vi "FPGAmain_5160_old.vi"() -> ()   [LabVIEW 2013]
uses:
  <vilib>/eio/EIONode/EIONode.xnode
  <vilib>/Platform/TimedLoop/XDataNode/wakeup.ctl
  <vilib>/Platform/TimedLoop/XDataNode/XDNodeRunTimeDep.lvlib
  <vilib>/Platform/TimedLoop/XDataNode/nitl_modes.ctl
  <vilib>/Platform/TimedLoop/XDataNode/timing_clust.ctl
  <vilib>/Platform/TimedLoop/XDataNode/XDataNode.xnode
  <vilib>/rvi/DataTransferAndStorage/Container/XNode/niFpgaContainer.xnode
  <vilib>/rvi/FIFO/Fifo_Resource/nirvififoEmulationWrite.vi
  <vilib>/rvi/FIFO/Fifo_Resource/nirvififoEmulationRead.vi
  <vilib>/rvi/interface/RandomDataEmulation/nirviRandomDataFpgaMultiElementTemplate.vi
  FPGA/AcquireState.ctl
  <instrlib>/FlexRIO/Libraries/Helper VIs/Counters/NI FlexRIO Counters.lvlib
  <instrlib>/FlexRIO/Libraries/Helper VIs/NI FlexRIO Helper VIs.lvlib
  <vilib>/rvi/FIFO/Fifo_Resource/nirvififoEmulationP2P.vi
  <vilib>/rvi/eio/common/nirviEmuTemplateMethod_errors.vi
  <vilib>/rvi/interface/RandomDataEmulation/nirviRandomDataFpgaReadWriteTemplate.vi
  FPGA/DataMode.ctl
panel:
  out "num data 2nd loop":u32
  out "timeout counter":i32
  out "num read":u32
  out "num to clock fifo":u32
  in  "Samples Per Trigger":i32 min=1 step=1
  in  "Trigger simulated data":bool
  in  "simulated phase":fxp<+,64,64>
  out "DMA Timed Out?":bool
  in  "phase":fxp<+,64,64>
  in  "Mode":T1
  in  "User Command Commit":bool
  in  "User Command":u8
  out "User Command Idle":bool
  out "User Command Status":u8
  in  "User Data 0":u16
  in  "User Data 1":u8
  out "PLL Locked":bool
  out "User Error":bool
  out "Configured?":bool
  # "Configuration"
  # "Aqcuistion"
  # "Simulated IQ"
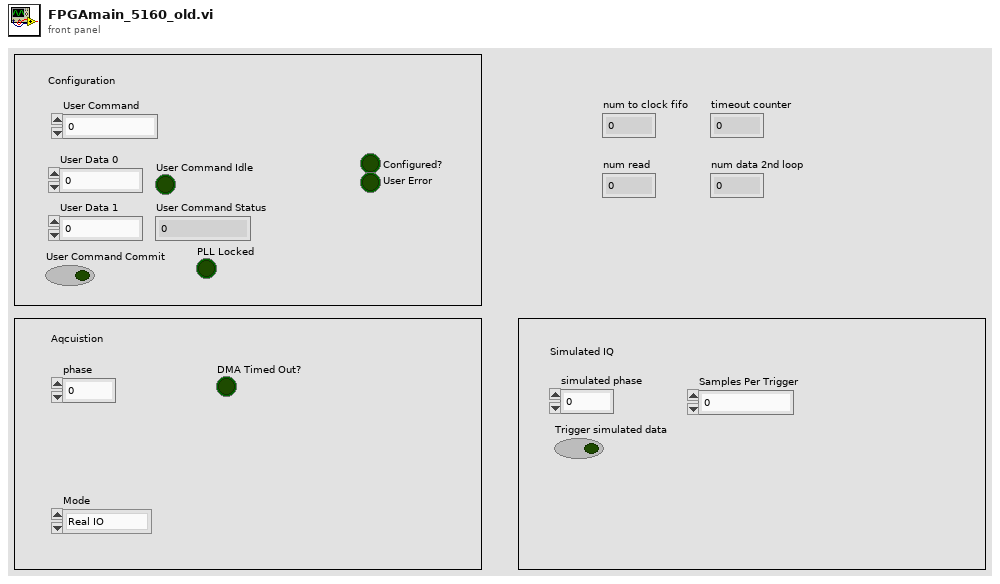
[diagram p1: front panel]
types:
  T1 = typedef "DataMode.ctl" = enum16{"Real IO", "Simulated"}
  T2 = typedef "AcquireState.ctl" = enum8{"Idle", "Acquire"}
  T3 = typedef "XDNodeRunTimeDep.lvlib/timing_clust.ctl" = cluster{"Expected End [f-1]":u64, "Actual End [f-1]":u64, "Finished Late? [f-1]":bool, "Expected End [i-1]":u64, "Actual End [i-1]":u64, "Finished Late? [i-1]":bool, "Expected Start [i]":u64, "Actual Start [i]":u64, "Expected Start [f]":u64, "Actual Start [f]":u64, "Source Name":string, "Structure Name":string, "Period":i64, "Deadline":i64, "Offset":i64, "Start":i64, "Priority":i32, "Timeout":i32, "Mode":T4, "Wakeup Reason":T5, "Error":errorcluster, "Source Type":string, "Secondary Source Type":string, "Global End Time":u64, "Global Start Time":u64, "Frame Duration":u64, "Iteration Duration":u64, "Assigned CPU":i32, "I/O Scan Engine Mode":u32}
  T4 = typedef "XDNodeRunTimeDep.lvlib/nitl_modes.ctl" = enum32{"No Change", "Process missed periods, maintain original phase", "Discard missed periods, maintain original phase", "Process missed periods, ignore original phase", "Discard missed periods, ignore original phase"}
  T5 = typedef "XDNodeRunTimeDep.lvlib/wakeup.ctl" = enum32{"Normal", "Aborted", "Asynchronous wakeup", "Timing source error", "Timed loop error", "Timeout"}
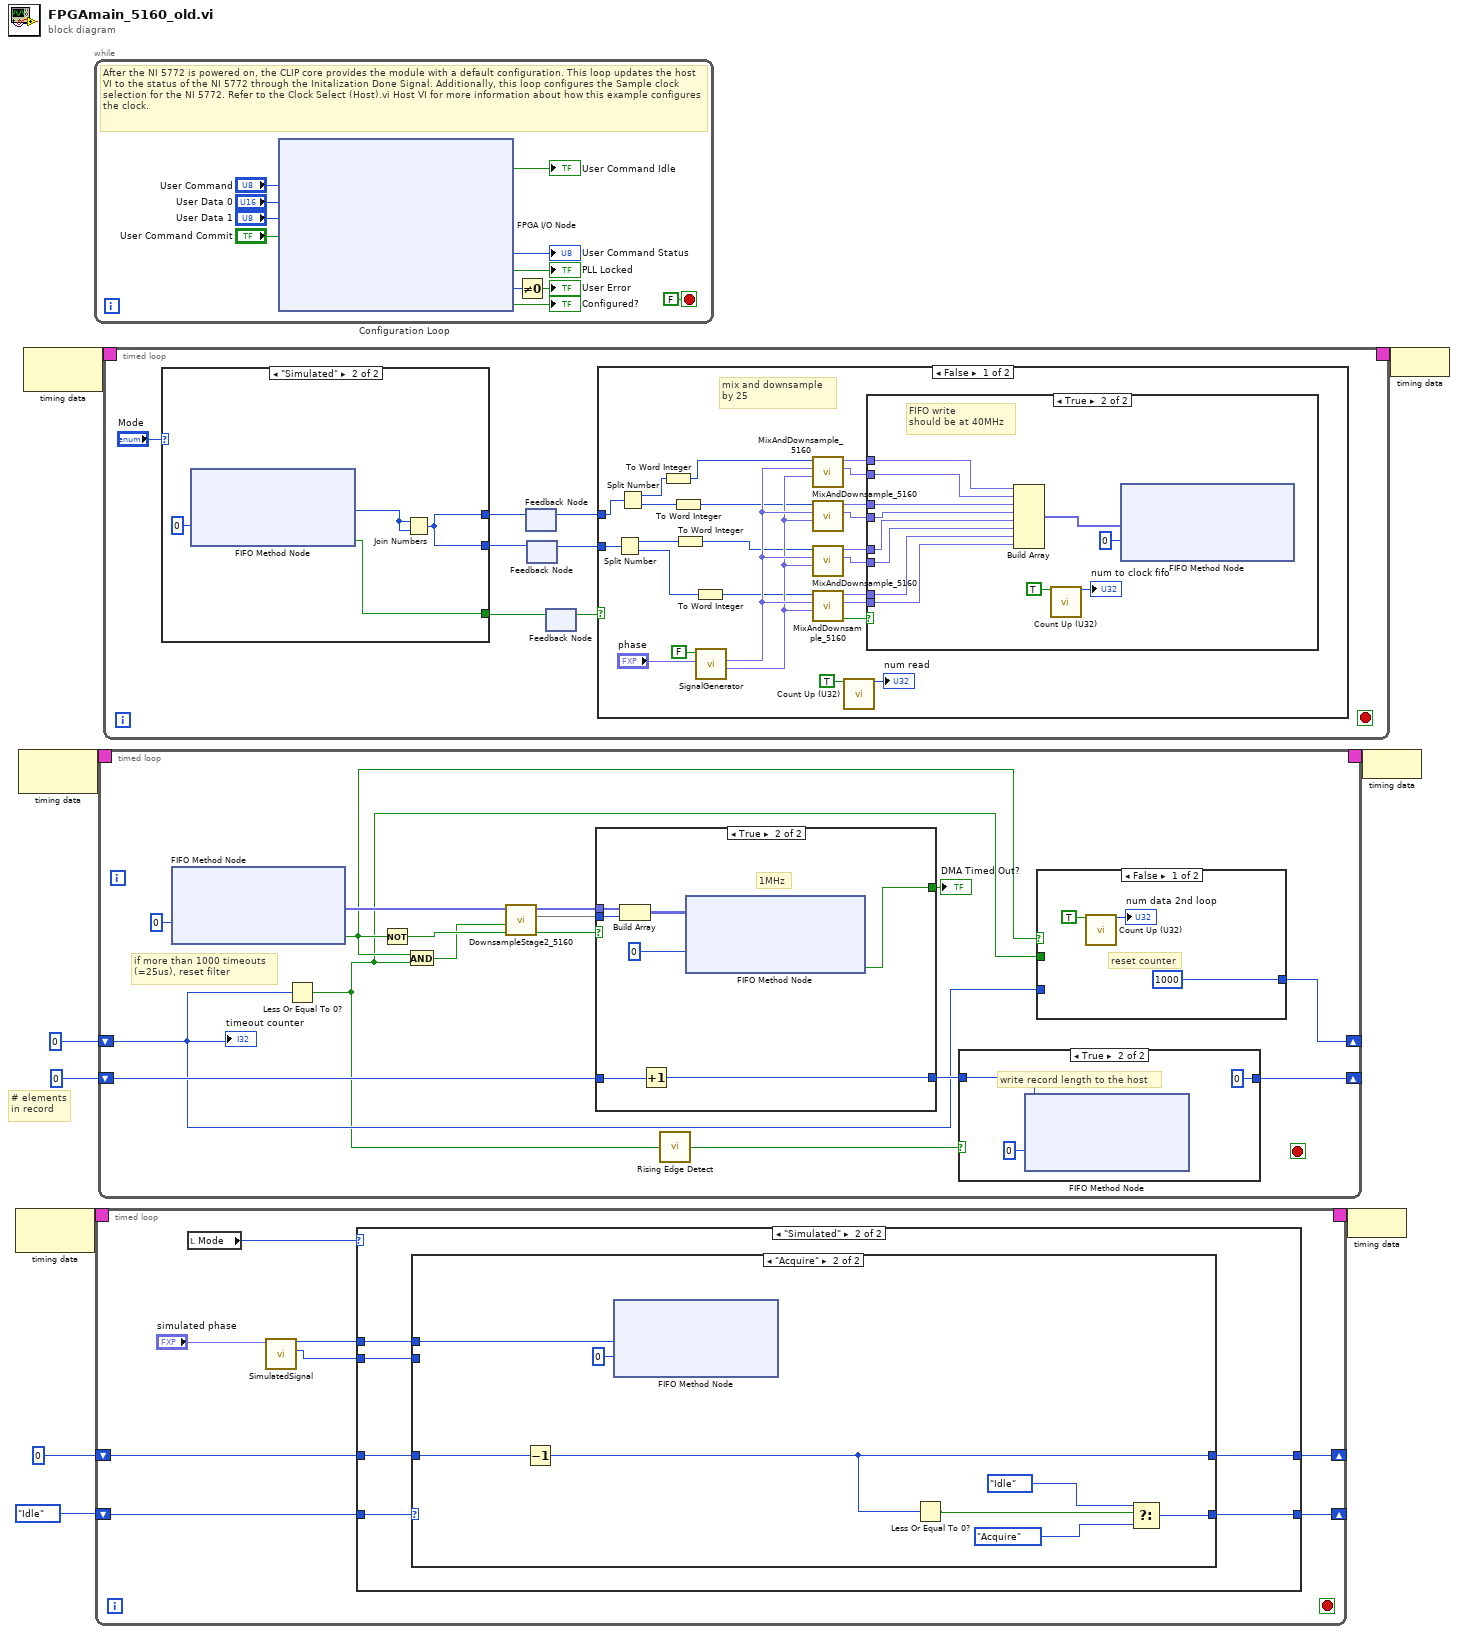
[diagram p0: block diagram]
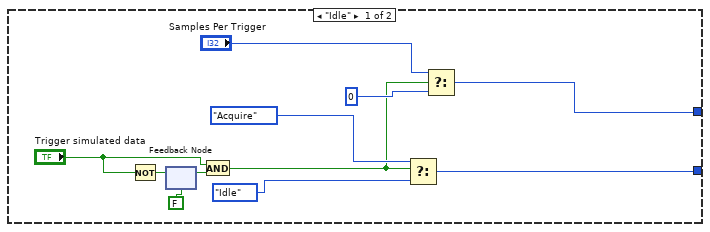
[diagram p3: hidden frame]
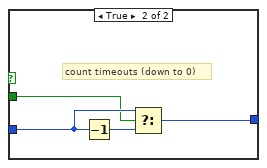
[diagram p4: hidden frame]
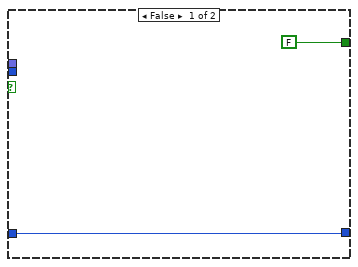
[diagram p6: hidden frame]
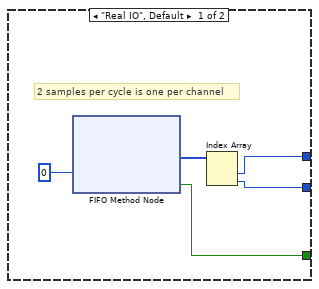
[diagram p9: hidden frame]
diagram:
  # "# elements\nin record"
  n1 = node-c288() -> (w6:T3)  [unwired: 1 in]
  n2 = node-c288() -> (w8:T3)  [unwired: 1 in]
  n3 = node-c288() -> (w10:T3)  [unwired: 1 in]
  n4 = while "Configuration Loop" {
    stop <- FALSE stop-if-true
    # "After the NI 5772 is powered on, the CLIP core provides the module with a default configuration. This loop updates the host VI to the status of the NI 5772 through the Initalization Done Signal. Additionally, this loop configures the Sample clock selection for the NI 5772. Refer to the Clock Select (Host).vi Host VI for more information about how this example configures the clock."
    n5 = xnode "FPGA I/O Node"("IO Module\\User Command"="User Command", "IO Module\\User Data 0"="User Data 0", "IO Module\\User Data 1"="User Data 1", "IO Module\\User Command Commit"="User Command Commit") -> ("IO Module\\User Command Idle"=→"User Command Idle":bool, "IO Module\\User Command Status"=→"User Command Status":u8, "IO Module\\PLL Locked"=→"PLL Locked":bool, "IO Module\\User Error"=w16:u8, "IO Module\\Initialization Done"=→"Configured?":bool)  [unwired: 9 in, 9 out]
    n6 = Not Equal To 0?(x=w16) -> (x != 0?=→"User Error":bool)
  }
  n7 = timed-loop {
    timing: w6 -> [_]
    timing-out: [_] -> w5
    shift-right: [w25] -> _
    shift-left: 0 ("f") -> [w24]
    shift-right: [w23] -> _
    shift-left: AcquireState."Idle" ("Acquire State") -> [w22]
    stop <- _ stop-if-true
    n8 = local read "Mode"() -> (w29:T1)
    n9 = call "SimulatedSignal.vi"("phase"="simulated phase") -> ("cos output"=w27:i16, "Sample output"=w28:i16)  [unwired: 9 in]
    n10 = case shown="\"Simulated\"" w29 {
      tunnel: w28 -> [_ w37]
      tunnel: w27 -> [_ w32]
      tunnel: [w31 w36] -> w25
      tunnel: w24 -> [w31 w35]
      tunnel: [w30 w34] -> w23
      tunnel: w22 -> [w30 w33]
      frame "Real IO" {
      }
      frame "Simulated" {
        n11 = case shown="\"Acquire\"" w33 {
          tunnel: w35 -> [_ w53]
          tunnel: [w42 w52] -> w34
          tunnel: [w39 w51] -> w36
          tunnel: w37 -> [_ w50]
          tunnel: w32 -> [_ _]
          frame "Idle" {
            n12 = Not(x="Trigger simulated data") -> (.not. x?=w43:bool)
            n13 = feedback #1(FALSE) -> (w44:bool)
            n14 = feedback-in #1(w43) -> ()
            n15 = And(x="Trigger simulated data", y=w44) -> (x .and. y?=w38:bool)
            n16 = Select(t=AcquireState."Acquire" ("Acquire State"), s=w38, f=AcquireState."Idle" ("Acquire State")) -> (s? t:f=w42:T2)
            n17 = Select(t="Samples Per Trigger", s=w38, f=0) -> (s? t:f=w39:i32)
          }
          frame "Acquire" {
            n18 = Decrement(x=w53) -> (x-1=w51:i32)
            n19 = xnode ("FIFO Method Node")("Element"=w50, "Timeout"=0) -> ()  [unwired: 1 in, 2 out]
            n20 = Less Or Equal To 0?(x=w51) -> (x <= 0?=w55:bool)
            n21 = Select(t=AcquireState."Idle" ("Acquire State"), s=w55, f=AcquireState."Acquire" ("Acquire State")) -> (s? t:f=w52:T2)
          }
        }
      }
    }
  }
  n22 = timed-loop {
    timing: w8 -> [_]
    timing-out: [_] -> w7
    shift-right: [w62] -> _
    shift-left: 0 ("y") -> [w61]
    shift-right: [w64] -> _
    shift-left: 0 ("y") -> [w66]
    stop <- _ stop-if-true
    # "if more than 1000 timeouts\n(=25us), reset filter"
    n23 = xnode ("FIFO Method Node")("Timeout"=0) -> ("Element"=w71:fxp<+/-,16,14>[], "Timed Out?"=w63:bool)  [unwired: 1 in, 1 out]
    n24 = Less Or Equal To 0?(x=w61) -> (x <= 0?=w60:bool)
    n25 = Not(x=w63) -> (.not. x?=w72:bool)
    n26 = And(x=w63, y=w60) -> (x .and. y?=w67:bool)
    n27 = call "DownsampleStage2_5160.vi"("valid in"=w72, "reset"=w67, "Element"=w71) -> ("valid out"=w73:bool, 2:w70, "Array"=w74:fxp<+/-,16,14>[])  [unwired: 6 in]
    n28 = case shown="True" w73 {
      tunnel: w74 -> [_ w93]
      tunnel: [FALSE ("Timed Out?") w91] -> w68
      tunnel: w70 -> [_ w92]
      tunnel: w66 -> [w86 w89]
      tunnel: [w86 w88] -> w65
      frame False {
      }
      frame True {
        # "1MHz"
        n29 = Build Array(w93, w92) -> (w90:fxp<+/-,16,14>[][])
        n30 = Increment(x=w89) -> (x+1=w88:i32)
        n31 = xnode ("FIFO Method Node")("Element"=w90, "Timeout"=0) -> ("Timed Out?"=w91:bool)  [unwired: 1 in, 1 out]
      }
    }
    "DMA Timed Out?" <- w68
    n32 = call <instrlib>:"Rising Edge Detect.vi"("signal"=w60) -> ("edge detected"=w59:bool)  [unwired: 14 in]
    n33 = case shown="True" w59 {
      tunnel: w65 -> [w82 w83]
      tunnel: [w82 0 ("y")] -> w64
      frame False {
      }
      frame True {
        # "write record length to the host"
        n34 = xnode ("FIFO Method Node")("Element"=w83, "Timeout"=0) -> ()  [unwired: 1 in, 2 out]
      }
    }
    n35 = case shown="False" w63 {
      tunnel: w60 -> [_ w79]
      tunnel: w61 -> [_ w80]
      tunnel: [1000 ("y") w78] -> w62
      frame False {
        # "reset counter"
        n36 = call <instrlib>:"Count Up (U32).vi"("increment"=TRUE) -> ("count out"=→"num data 2nd loop":u32)  [unwired: 14 in]
      }
      frame True {
        # "count timeouts (down to 0)"
        n37 = Decrement(x=w80) -> (x-1=w81:i32)
        n38 = Select(t=w80, s=w79, f=w81) -> (s? t:f=w78:i32)
      }
    }
    "timeout counter" <- w61
  }
  n39 = timed-loop {
    timing: w10 -> [_]
    timing-out: [_] -> w9
    stop <- _ stop-if-true
    n40 = case shown="\"Simulated\"" "Mode" {
      tunnel: [w143 w147] -> w102
      tunnel: [w141 w148] -> w99
      tunnel: [w142 w147] -> w98
      frame "Real IO", Default {
        # "2 samples per cycle is one per channel"
        n41 = xnode ("FIFO Method Node")("Timeout"=0) -> ("Element"=w145:u32[], "Timed Out?"=w141:bool)  [unwired: 1 in, 1 out]
        n42 = Index Array(array=w145) -> (element #1=w143:u32, element #2=w142:u32)  [unwired: 2 in]
      }
      frame "Simulated" {
        n43 = xnode ("FIFO Method Node")("Timeout"=0) -> ("Element"=w146:i16, "Timed Out?"=w148:bool)  [unwired: 1 in, 1 out]
        n44 = Join Numbers(hi=w146, lo=w146) -> ((hi.lo)=w147:u32)
      }
    }
    n45 = feedback-in #2(w102) -> ()
    n46 = feedback #2() -> (w101:u32)  [unwired: 1 in]
    n47 = feedback #3() -> (w97:u32)  [unwired: 1 in]
    n48 = feedback-in #3(w98) -> ()
    n49 = feedback #4() -> (w100:bool)  [unwired: 1 in]
    n50 = feedback-in #4(w99) -> ()
    n51 = case shown="False" w100 {
      tunnel: w101 -> [w119 _]
      tunnel: w97 -> [w108 _]
      frame False {
        # "mix and downsample\nby 25"
        n52 = Split Number(x=w108) -> (hi(x)=w109:u16, lo(x)=w110:u16)
        n53 = Split Number(x=w119) -> (hi(x)=w118:u16, lo(x)=w117:u16)
        n54 = To Word Integer(number=w118) -> (16bit integer=w112:i16)
        n55 = To Word Integer(number=w117) -> (16bit integer=w111:i16)
        n56 = To Word Integer(number=w109) -> (16bit integer=w106:i16)
        n57 = To Word Integer(number=w110) -> (16bit integer=w107:i16)
        n58 = call "SignalGenerator.vi"("phase"="phase", "Reset"=FALSE) -> ("Cos"=w113:fxp<+/-,16,0>, "Sin"=w114:fxp<+/-,16,0>)  [unwired: 7 in, 1 out]
        n59 = call "MixAndDownsample_5160.vi"("Sine in"=w113, "Cosine in"=w114, "Sample in"=w112) -> ("Q out"=w126:fxp<+/-,16,14>, "I out"=w128:fxp<+/-,16,14>)  [unwired: 6 in, 1 out]
        n60 = call "MixAndDownsample_5160.vi"("Sine in"=w113, "Cosine in"=w114, "Sample in"=w111) -> ("Q out"=w124:fxp<+/-,16,14>, "I out"=w125:fxp<+/-,16,14>)  [unwired: 6 in, 1 out]
        n61 = call "MixAndDownsample_5160.vi"("Sine in"=w113, "Cosine in"=w114, "Sample in"=w106) -> ("Q out"=w122:fxp<+/-,16,14>, "I out"=w123:fxp<+/-,16,14>)  [unwired: 6 in, 1 out]
        n62 = call "MixAndDownsample_5160.vi"("Sine in"=w113, "Cosine in"=w114, "Sample in"=w107) -> ("valid out"=w127:bool, "Q out"=w120:fxp<+/-,16,14>, "I out"=w121:fxp<+/-,16,14>)  [unwired: 6 in]
        n63 = call <instrlib>:"Count Up (U32).vi"("increment"=TRUE) -> ("count out"=→"num read":u32)  [unwired: 14 in]
        n64 = case shown="True" w127 {
          tunnel: w128 -> [_ w139]
          tunnel: w126 -> [_ w138]
          tunnel: w125 -> [_ w137]
          tunnel: w124 -> [_ w131]
          tunnel: w123 -> [_ w136]
          tunnel: w122 -> [_ w135]
          tunnel: w121 -> [_ w134]
          tunnel: w120 -> [_ w133]
          frame False {
          }
          frame True {
            # "FIFO write\nshould be at 40MHz"
            n65 = Build Array(w139, w138, w137, w131, w136, w135, w134, w133) -> (w132:fxp<+/-,16,14>[])
            n66 = call <instrlib>:"Count Up (U32).vi"("increment"=TRUE) -> ("count out"=→"num to clock fifo":u32)  [unwired: 14 in]
            n67 = xnode ("FIFO Method Node")("Element"=w132, "Timeout"=0) -> ()  [unwired: 1 in, 2 out]
          }
        }
      }
      frame True {
        # "FIFO read timeout, no data"
      }
    }
  }
  n68 = node-c288(w5) -> ()
  n69 = node-c288(w7) -> ()
  n70 = node-c288(w9) -> ()
